vi "Emergency Fatal Error.vi"(8 "error in (no error)":errorcluster, 10 "Error":string, 11 "SCADA in":refnum<class "SCADA.lvclass">) -> (0 "error out":errorcluster, 3 "SCADA out":refnum<class "SCADA.lvclass">)   [LabVIEW 2015, in "SCADA Core.lvlib" / "SCADA.lvclass"]
uses:
  SCADA.lvclass
  <vilib>/ActorFramework/Message Enqueuer/Message Priority.ctl
  <vilib>/ActorFramework/Actor/Actor.lvclass/Actor.ctl
  <vilib>/ActorFramework/Message Enqueuer/Message Enqueuer.lvclass/Message Enqueuer.ctl
  SCADA.lvclass/SCADA.ctl
  <vilib>/ActorFramework/Message Enqueuer/Init from Existing Queue.vi
  <vilib>/ActorFramework/Message Enqueuer/Enqueue.vi
  <vilib>/ActorFramework/Message Priority Queue/Priority Enqueue.vi
  <vilib>/ActorFramework/Message Enqueuer/Message Enqueuer.lvclass
  SCADA Action Messages/Shutdown Msg/Shutdown Msg.lvclass
  <vilib>/ActorFramework/Actor/Actor.lvclass
  SCADA Abstract Messages/Emergency Status Msg/Emergency Status Msg.lvclass
  Utilities/Message Strings.llb/Message String Utilities.lvlib
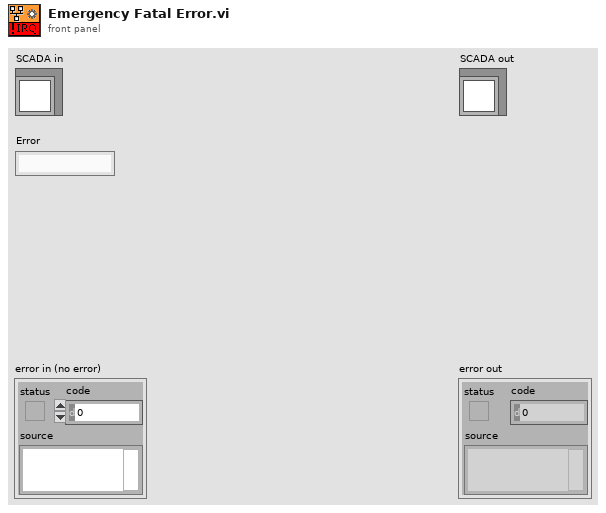
[diagram p1: front panel]
types:
  T1 = typedef "Actor Framework.lvlib/Message Enqueuer.lvclass/Message Priority.ctl" = enum16{"Low", "Normal", "High"}
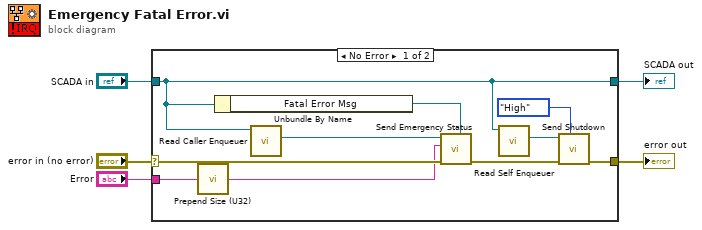
[diagram p0: block diagram]
diagram:
  n1 = case shown="No Error" "error in (no error)" {
    selector: "error in (no error)" -> [w13 w17]
    tunnel: [w9 w17] -> w4
    tunnel: [w7 w16] -> w2
    tunnel: "SCADA in" -> [w7 w16]
    tunnel: "Error" -> [w12 _]
    frame No Error {
      n2 = call "Prepend Size (U32).vi"("String in"=w12) -> ("String out"=w11:string)
      n3 = Unbundle By Name(w7) -> ("Fatal Error Msg"=w15:refnum<class "Emergency Status Msg.lvclass">)
      n4 = call <vilib>:"Read Caller Enqueuer.vi"("Actor"=w7) -> ("Caller Enqueuer"=w14:refnum<class "Message Enqueuer.lvclass">)  [unwired: 10 in]
      n5 = call "Send Emergency Status.vi"("Emergency Status Msg"=w15, "error in (no error)"=w13, "content"=w11, "Message Enqueuer in"=w14) -> ("error out"=w10:errorcluster)  [unwired: 6 in, 1 out]
      n6 = call <vilib>:"Read Self Enqueuer.vi"("Actor"=w7) -> ("Self Enqueuer"=w8:refnum<class "Message Enqueuer.lvclass">)  [unwired: 10 in]
      n7 = call "Send Shutdown.vi"("Message Priority (Normal)"=Message_Priority."High", "error in (no error)"=w10, "Message Enqueuer"=w8) -> ("error out"=w9:errorcluster)  [unwired: 7 in, 1 out]
    }
    frame Error {
    }
  }
  "error out" <- w4
  "SCADA out" <- w2
